vi "PlotVisibilityCheckbox.vi"() -> ()   [LabVIEW 2013]
doc: "This VI show how to control waveform visibility of waveform graph."
uses:
  <vilib>/measure/NI_MABase.lvlib
panel:
  out "Waveform Graph":waveform(dbl)[](graph)
  # "Visible Items->Plot Visibility Checkbox"
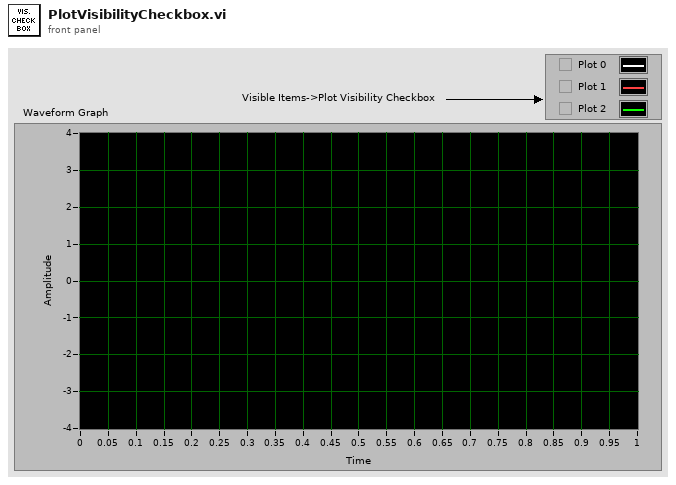
[diagram p1: front panel]
types:
  T1 = enum16{"Sine Wave", "Triangle Wave", "Square Wave", "Sawtooth Wave"}
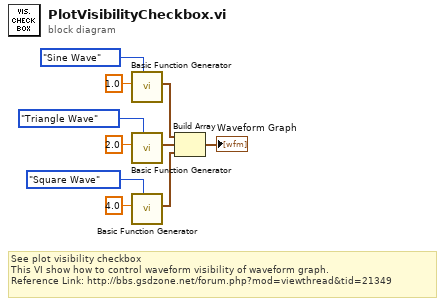
[diagram p0: block diagram]
diagram:
  # "See plot visibility checkbox\nThis VI show how to control waveform visibility of waveform graph.\nReference Link: http://bbs.gsdzone.net/forum.php?mod=viewthread&tid=21349"
  n1 = call <vilib>:"Basic Function Generator.vi"("signal type"=T1."Sine Wave", "amplitude"=1.0) -> ("signal out"=w7:waveform(dbl))  [unwired: 7 in, 2 out]
  n2 = call <vilib>:"Basic Function Generator.vi"("signal type"=T1."Triangle Wave", "amplitude"=2.0) -> ("signal out"=w6:waveform(dbl))  [unwired: 7 in, 2 out]
  n3 = call <vilib>:"Basic Function Generator.vi"("signal type"=T1."Square Wave", "amplitude"=4.0) -> ("signal out"=w5:waveform(dbl))  [unwired: 7 in, 2 out]
  n4 = Build Array(w7, w6, w5) -> (→"Waveform Graph":waveform(dbl)[])
